vi "Get Data Log File Span Settings.vi"(8 "error in":errorcluster, 11 "File Ref In":T2 format="%.0x") -> (0 "error out":errorcluster, 1 "Segment Size":u32, 2 "Segment Files By":T1, 3 "File Ref Out":T2 format="%.0x", 4 "Segment Files":bool)   [LabVIEW 2019, in "Embedded Data Logger Shared.lvlib"]
uses:
  Embedded Data Logger Shared.lvlib
  <vilib>/NI VeriStand/Custom Device API/Custom Device Item Ref.ctl
  Segment Files By.ctl
  Constants.vi
  <vilib>/NI VeriStand/Custom Device API/Get Item Property (U32).vi
  <vilib>/NI VeriStand/Custom Device API/Get Item Property (Boolean).vi
  <vilib>/NI VeriStand/Custom Device API/Get Item Property (U16).vi
  <vilib>/NI VeriStand/Custom Device API/Custom Device API.lvlib
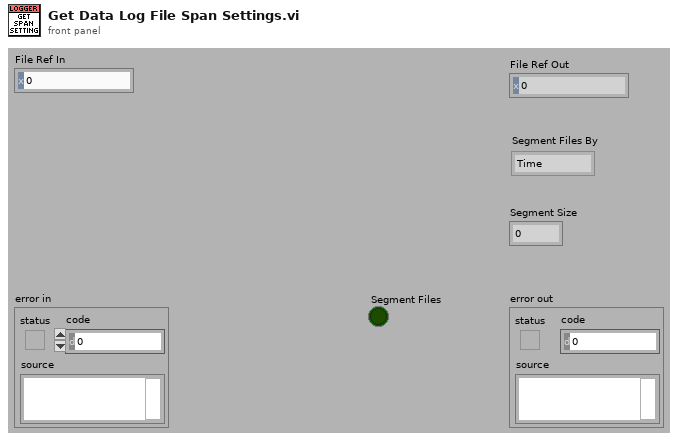
[diagram p1: front panel]
types:
  T1 = typedef "Embedded Data Logger Shared.lvlib/Segment Files By.ctl" = enum16{"Time", "Size"}
  T2 = typedef "Custom Device API.lvlib/Custom Device Item Ref.ctl" = u64
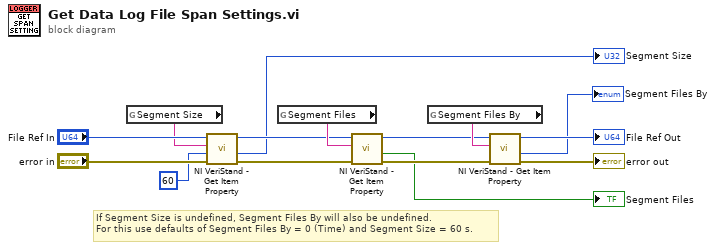
[diagram p0: block diagram]
diagram:
  # "If Segment Size is undefined, Segment Files By will also be undefined.\nFor this use defaults of Segment Files By = 0 (Time) and Segment Size = 60 s."
  n1 = global read "Constants.vi" "Segment Size"() -> (w13:string)
  n2 = call-poly <vilib>:"NI VeriStand - Get Item Property.vi"("error in (no error)"="error in", "Default Value"=u32 60, "Property Name"=w13, "Item Ref in"="File Ref In") -> ("error out"=w8:errorcluster, "Value"=→"Segment Size":u32, "Item Ref out"=w9:T2)  [unwired: 5 out]
  n3 = global read "Constants.vi" "Segment Files"() -> (w12:string)
  n4 = call-poly <vilib>:"NI VeriStand - Get Item Property.vi"("error in (no error)"=w8, "Property Name"=w12, "Item Ref in"=w9) -> ("error out"=w4:errorcluster, "Value"=→"Segment Files":bool, "Item Ref out"=w5:T2)  [unwired: 1 in, 5 out]
  n5 = global read "Constants.vi" "Segment Files By"() -> (w7:string)
  n6 = call-poly <vilib>:"NI VeriStand - Get Item Property.vi"("error in (no error)"=w4, "Property Name"=w7, "Item Ref in"=w5) -> ("error out"=→"error out":errorcluster, "Value"=→"Segment Files By":u16, "Item Ref out"=→"File Ref Out":T2)  [unwired: 1 in, 5 out]
